vi "CODMn插入数据.vi"(0 "database":string, 1 "data":T2 {"单位" items=["ug/L", "mg/L", "ppm", "mg/m3", "cm", "ppb", "ug/m3", "%", "nmol/mol", "umol/mol", "MPN/L", "MPN/100ml", "ng/m3", "NTU", "无量纲", "ms/cm", "us/cm"]}, 3 "SN":string, 5 "table":string, 7 "测量模式":T3(ring)=enum."水样测试", 9 "数据类型":string(combo)="N", 11 "error in (no error)":errorcluster) -> (15 "error out":errorcluster)   [LabVIEW 2016, in "斯坦道CODMn新电路板.lvlib"]
uses:
  <vilib>/Utility/sysdir.llb/System Directory Type.ctl
  <vilib>/Utility/error.llb/DialogType.ctl
  <vilib>/addons/database/Auxilliary.llb/DB Tools Column Info.ctl
  <vilib>/addons/database/Auxilliary.llb/DB Tools DataTypes.ctl
  <vilib>/addons/database/Connection.llb/DB Tools Open Connec (String).vi
  <vilib>/addons/database/Connection.llb/Conn Execute.vi
  <vilib>/addons/database/Recordset.llb/Rec Fetch Recordset Data (R).vi
  <vilib>/addons/database/Recordset.llb/Rec Destroy - Connection.vi
  <vilib>/addons/database/NI_Database_API.lvlib
  <vilib>/Utility/VariantDataType/VariantType.lvlib
panel:
  out "data输出":T1
  out "为空？":bool
  out "recordset data":variant[][](array[variant])
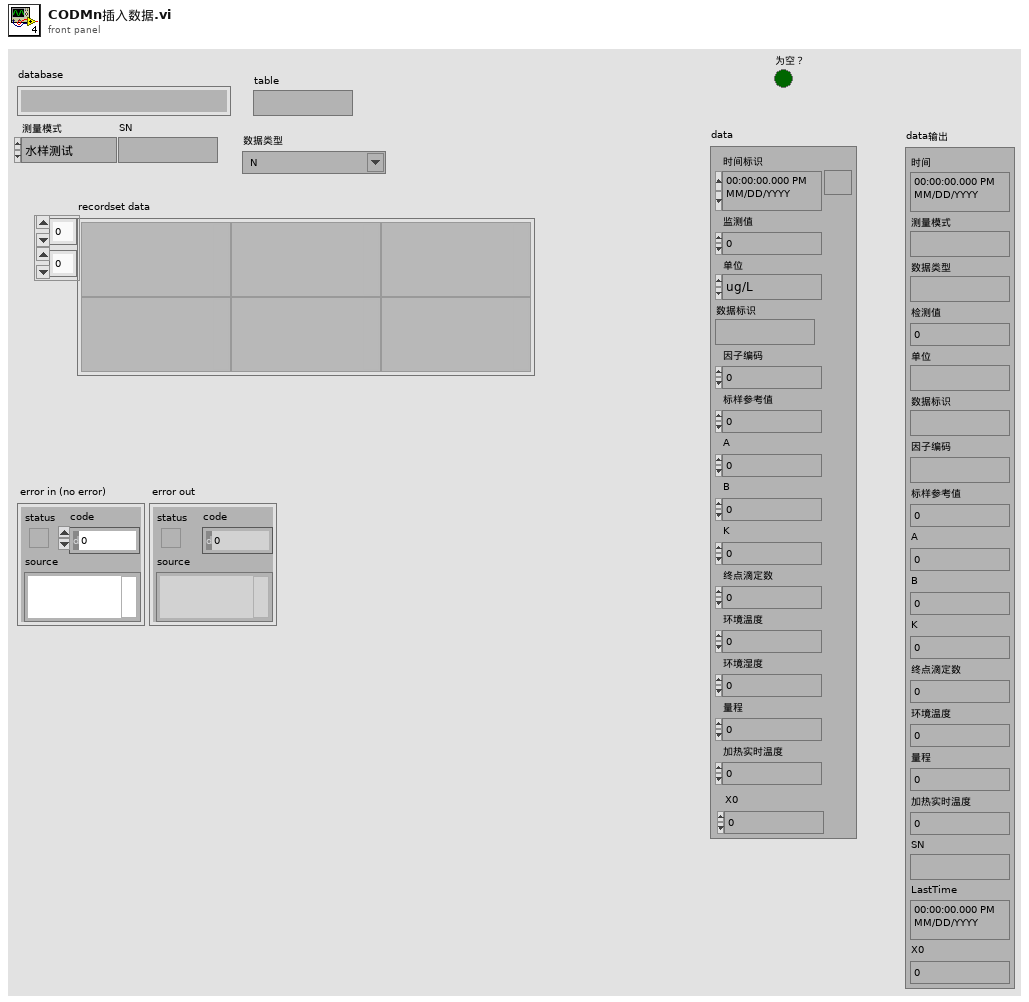
[diagram p1: front panel]
types:
  T1 = cluster{"时间":timestamp, "测量模式":string, "数据类型":string, "检测值":sgl, "单位":string, "数据标识":string, "因子编码":string, "标样参考值":sgl, "A":sgl, "B":sgl, "K":sgl, "终点滴定数":sgl, "环境温度":sgl, "量程":sgl, "加热实时温度":sgl, "SN":string, "LastTime":timestamp, "X0":sgl}
  T2 = cluster{"时间标识":timestamp, "监测值":sgl, "单位":u16, "数据标识":string, "因子编码":u32, "标样参考值":sgl, "A":sgl, "B":sgl, "K":sgl, "终点滴定数":sgl, "环境温度":sgl, "环境湿度":sgl, "量程":sgl, "加热实时温度":sgl, "X0":sgl}
  T3 = enum16{"维护数据", "水样测试", "标样核查", "零点核查", "跨度核查", "空白测试", "平行样测试", "加标回收", "空白校准", "标样校准", "初始化（清洗）"}
  T4 = typedef "DialogType.ctl" = u16
  T5 = typedef "System Directory Type.ctl" = i32
  T6 = typedef "NI_Database_API.lvlib/Conn ObjectReference.ctl" = refnum<k1>
  T7 = typedef "NI_Database_API.lvlib/Rec ObjectReference.ctl" = refnum<k1>
  T8 = typedef "NI_Database_API.lvlib/DB Tools Column Info.ctl" = cluster{"column name":string, "data type":T9, "size":i32, "allow null?":bool}
  T9 = typedef "NI_Database_API.lvlib/DB Tools DataTypes.ctl" = enum16{"String", "Long (I32)", "Single (SGL)", "Double (DBL)", "Date/Time", "Binary"}
  T10 = cluster{"测量量程":dbl, "测量精度":dbl, "测量间隔":dbl, "消解温度":dbl, "消解时长":dbl, "空白校准时间":timestamp, "曲线截距":dbl, "曲线斜率":dbl, "测量检出限":dbl, "测量信号值":dbl, "线性相关系数":dbl, "二次多项式系数":dbl, "标样校准时间":timestamp, "稀释倍数":dbl, "三项式系数":dbl, "空白标定系数":dbl, "量程系数":dbl, "F0/ORPA":dbl, "F1/ORPB":dbl, "F2/ORPK":dbl, "F3":dbl, "F4":dbl, "F5":dbl, "F6":dbl, "F7":dbl, "X0/滴定数":dbl, "量程":dbl}
  T11 = typedef "VariantType.lvlib/Type.ctl" = enum8{"Invalid Type", "Void", "I8", "I16", "I32", "I64", "U8", "U16", "U32", "U64", "Single Float", "Double Float", "Extended Float", "Single Complex", "Double Complex", "Extended Complex", "Enum U8", "Enum U16", "Enum U32", "Enum U64", "Single Float With Unit", "Double Float With Unit", "Extended Float With Unit", "Single Complex with Unit", "Double Complex with Unit", "Extended Complex with Unit", "Boolean", "String", "Path", "Picture", "Tag", "Array", "Cluster", "Variant", "LV Variant", "Waveform", "Timestamp", "Digital Waveform", "Digital Data", "ExpressData", "Refnum", "External Data", "VI", "Poly VI", "LabVIEW Class Instance", "Fixed Point"}
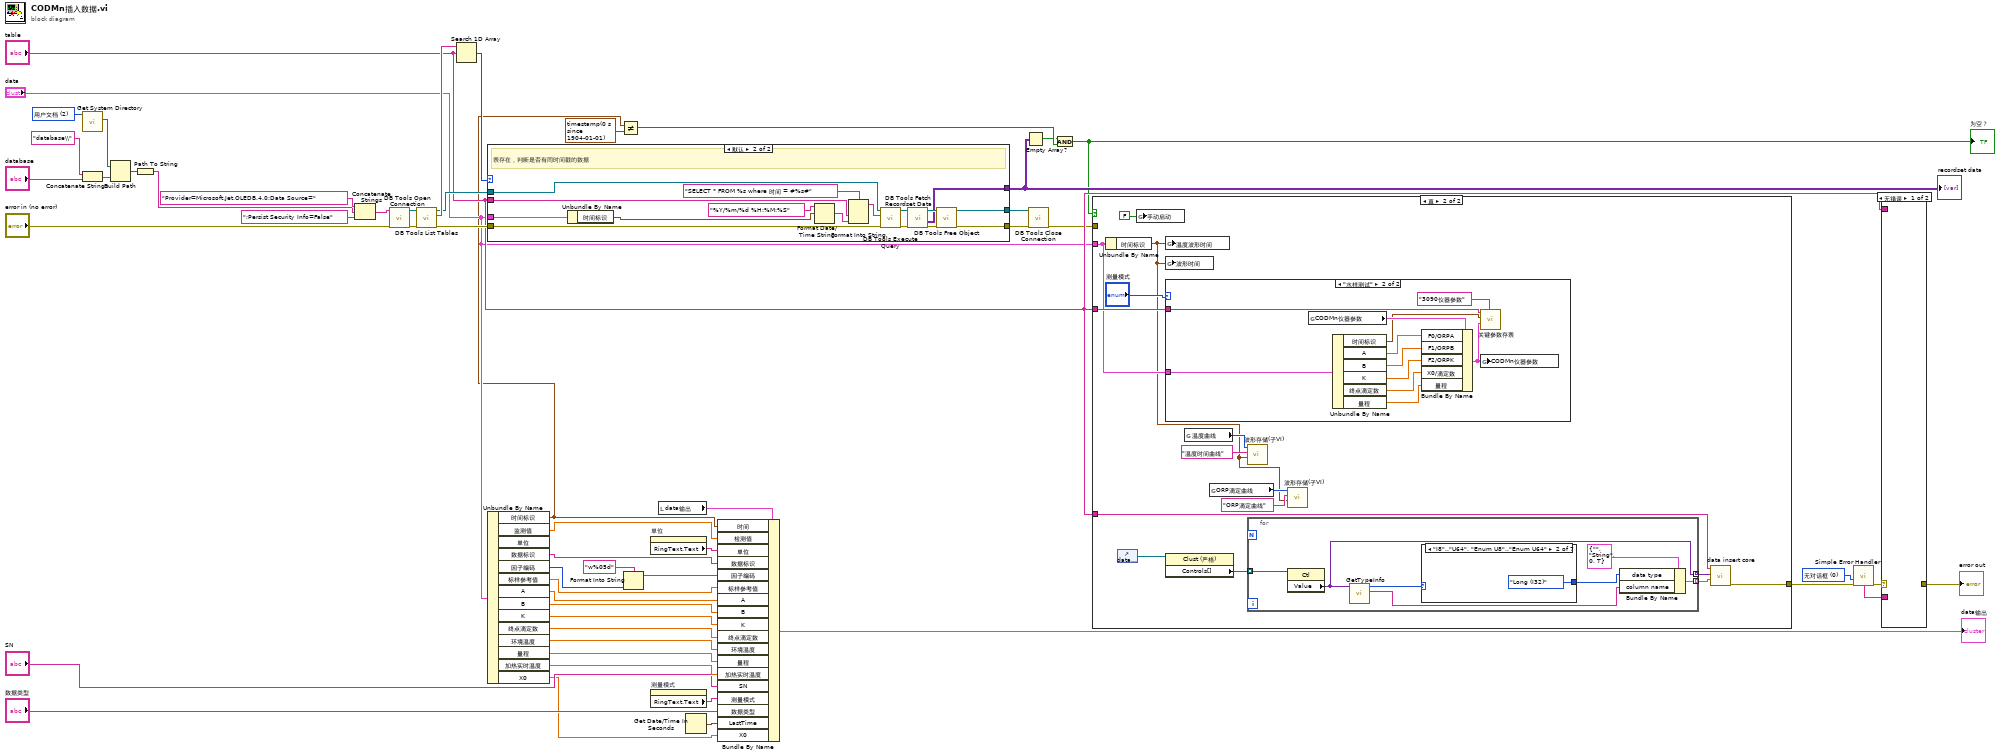
[diagram p0: block diagram]
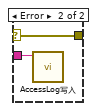
[diagram p2: hidden frame]
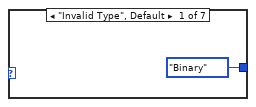
[diagram p4: hidden frame]
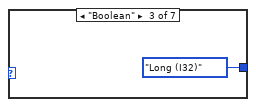
[diagram p5: hidden frame]
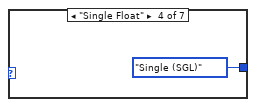
[diagram p6: hidden frame]
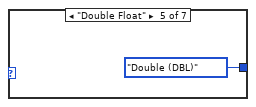
[diagram p7: hidden frame]
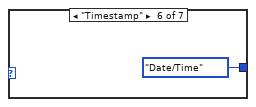
[diagram p8: hidden frame]
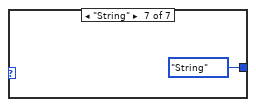
[diagram p9: hidden frame]
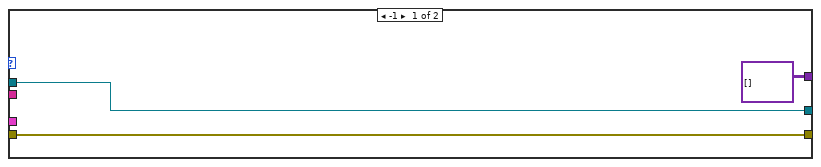
[diagram p11: hidden frame]
diagram:
  w36 = T4 0 items=["无对话框", "确定信息", "继续或停止信息", "确定信息＋警告", "继续/停止+警告"] ("type of dialog (OK msg:1)")
  w53 = T5 2 items=["用户目录"=0, "用户桌面"=1, "用户文档"=2, "用户应用程序数据"=3, "用户设置"=4, "用户临时目录"=5, "公共文档"=6, "公共应用程序数据"=7, "公共设置"=8, "公共缓存"=13, "系统核心库"=9, "系统安装库"=10, "应用程序文件"=11, "启动盘根目录"=12] ("system directory type")
  n1 = call <vilib>:"Get System Directory.vi"("system directory type"=w53) -> ("system directory"=w51:path)  [unwired: 10 in]
  n2 = Concatenate Strings("database\\" ("condition"), "database") -> (w45:string)
  n3 = Build Path(base path=w51, name or relative path=w45) -> (appended path=w50:path)
  n4 = Path To String(path=w50) -> (string=w49:string)
  n5 = Concatenate Strings("Provider=Microsoft.Jet.OLEDB.4.0;Data Source=" ("condition"), w49, ";Persist Security Info=False" ("condition")) -> (w47:string)
  n6 = call-poly <vilib>:"DB Tools Open Connection.vi"("error in (no error)"="error in (no error)", "connection information"=w47) -> ("error out"=w42:errorcluster, "connection reference"=w43:T6)  [unwired: 6 in]
  n7 = call <vilib>:"DB Tools List Tables.vi"("error in (no error)"=w42, "connection reference"=w43) -> ("error out"=w37:errorcluster, "tables"=w41:string[], "connection reference out"=w38:T6)  [unwired: 3 in]
  n8 = Search 1D Array(1D array=w41, element="table") -> (index of element=w40:i32)  [unwired: 1 in]
  n9 = case shown="默认" w40 {
    tunnel: [variant[][] [] ("recordset data") w69] -> w44
    tunnel: [w57 w68] -> w31
    tunnel: [w56 w67] -> w30
    tunnel: w38 -> [w57 w61]
    tunnel: w37 -> [w56 w60]
    tunnel: "table" -> [_ w59]
    tunnel: "data" -> [_ w62]
    frame -1 {
    }
    frame Default {
      # "表存在，判断是否有同时间戳的数据"
      n10 = Unbundle By Name(w62) -> ("时间标识"=w65:timestamp)
      n11 = Format Date/Time String(time format string (%c)="%Y/%m/%d %H:%M:%S" ("时间格式字符串(%c)"), seconds (now)=w65) -> (date/time string=w63:string)  [unwired: 1 in]
      n12 = Format Into String(format string="SELECT * FROM %s where 时间 = #%s#" ("格式字符串"), w59, w63) -> (resulting string=w66:string)  [unwired: 2 in, 1 out]
      n13 = call-poly <vilib>:"DB Tools Execute Query.vi"("error in (no error)"=w60, "SQL query"=w66, "connection reference"=w61) -> ("error out"=w70:errorcluster, "recordset reference"=w73:T7)  [unwired: 5 in]
      n14 = call-poly <vilib>:"DB Tools Fetch Recordset Data.vi"("error in (no error)"=w70, "recordset reference"=w73) -> ("error out"=w71:errorcluster, "recordset data"=w69:variant[][], "recordset reference out"=w72:T7)  [unwired: 3 in]
      n15 = call-poly <vilib>:"DB Tools Free Object.vi"("error in (no error)"=w71, "recordset reference"=w72) -> ("error out"=w67:errorcluster, "connection reference"=w68:T6)  [unwired: 8 in]
    }
  }
  "recordset data" <- w44
  n16 = Unbundle By Name("data") -> ("时间标识"=w5:timestamp, "监测值"=w25:sgl, "数据标识"=w23:string, "因子编码"=w21:u32, "标样参考值"=w19:sgl, "A"=w18:sgl, "B"=w17:sgl, "K"=w16:sgl, "终点滴定数"=w15:sgl, "环境温度"=w14:sgl, "量程"=w13:sgl, "加热实时温度"=w12:sgl, "X0"=w7:sgl)  [unwired: 1 out]
  n17 = Not Equal?(x=w5, y=timestamp(0 s since 1904-01-01)) -> (x != y?=w3:bool)
  n18 = Format Into String(format string="w%05d" ("格式字符串"), w21) -> (resulting string=w20:string)  [unwired: 2 in, 1 out]
  n19 = property on="单位" class="Ring (严格)"() -> ("RingText.Text"=w24:string)  [unwired: 2 in, 2 out]
  n20 = property on="测量模式" class="Enum (严格)"() -> ("RingText.Text"=w10:string)  [unwired: 2 in, 2 out]
  n21 = local read "data输出"() -> (w28:T1)
  n22 = Get Date/Time In Seconds() -> (seconds since 1Jan1904=w8:timestamp)
  n23 = Bundle By Name(cluster=w28, "时间"=w5, "检测值"=w25, "单位"=w24, "数据标识"=w23, "因子编码"=w20, "标样参考值"=w19, "A"=w18, "B"=w17, "K"=w16, "终点滴定数"=w15, "环境温度"=w14, "量程"=w13, "加热实时温度"=w12, "SN"="SN", "测量模式"=w10, "数据类型"="数据类型", "LastTime"=w8, "X0"=w7) -> (→"data输出":T1)
  n24 = Empty Array?(array=w44) -> (empty?=w2:bool)
  n25 = call <vilib>:"DB Tools Close Connection.vi"("error in (no error)"=w30, "connection reference"=w31) -> ("error out"=w29:errorcluster)  [unwired: 5 in]
  n26 = And(x=w2, y=w3) -> (x .and. y?=w1:bool)
  "为空？" <- w1
  n27 = case shown="真" w1 {
    tunnel: "table" -> [_ w75]
    tunnel: "data" -> [_ w86]
    tunnel: w29 -> [_ _]
    tunnel: "table" -> [_ w88]
    tunnel: [_ w74] -> w6
    frame False {
    }
    frame True {
      n28 = Unbundle By Name(w86) -> ("时间标识"=w81:timestamp)
      n29 = control-ref of="data输出"() -> (w79:refnum<vi>)
      n30 = global write "VARCODMn全局变量.vi" "手动启动"(FALSE ("手动启动")) -> ()
      n31 = global write "VARCODMn全局变量.vi" "温度波形时间"(w81) -> ()
      n32 = global write "VARCODMn全局变量.vi" "波形时间"(w81) -> ()
      n33 = case shown="\"水样测试\"" "测量模式" {
        tunnel: w86 -> [_ w112]
        tunnel: w88 -> [_ w110]
        frame "维护数据", Default {
        }
        frame "水样测试" {
          n34 = global read "CODMn断电保存全局变量.vi" "CODMn仪器参数"() -> (w113:T10)
          n35 = Unbundle By Name(w112) -> ("时间标识"=w104:timestamp, "A"=w109:sgl, "B"=w108:sgl, "K"=w107:sgl, "终点滴定数"=w106:sgl, "量程"=w105:sgl)
          n36 = Bundle By Name(cluster=w113, "F0/ORPA"=w109, "F1/ORPB"=w108, "F2/ORPK"=w107, "X0/滴定数"=w106, "量程"=w105) -> (w103:T10)
          n37 = call "关键参数存表.vi"("table"="3090仪器参数", "仪器参数"=w103, "datatime"=w104, "仪器名称"=w110) -> ()  [unwired: 7 in, 1 out]
          n38 = global write "CODMn断电保存全局变量.vi" "CODMn仪器参数"(w103) -> ()
        }
      }
      n39 = property class="Clust (严格)"(reference=w79) -> ("Controls[]"=w77:refnum<vi>[])  [unwired: 1 in, 2 out]
      n40 = global read "VARCODMn全局变量.vi" "温度曲线"() -> (w83:u16[])
      n41 = global read "VARCODMn全局变量.vi" "ORP滴定曲线"() -> (w85:u16[])
      n42 = call "波形存储(子VI).vi"("波形时间"=w81, "condition"="温度时间曲线", "ORP滴定曲线"=w83) -> ()  [unwired: 9 in]
      n43 = for {
        tunnel: w77 -> [w95] mode=indexing
        tunnel: [w89] -> w78 mode=indexing
        tunnel: [w90] -> w76 mode=indexing
        n44 = property class="Ctl"(reference=w95) -> ("Value"=w89:variant)  [unwired: 1 in, 2 out]
        n45 = call <vilib>:"GetTypeInfo.vi"("Variant"=w89) -> ("Name"=w93:string, "Type Enum"=w92:T11)  [unwired: 6 in, 3 out]
        n46 = case shown="\"I8\"..\"U64\", \"Enum U8\"..\"Enum U64\"" w92 {
          tunnel: [DB_Tools_DataTypes."Binary" ("data type") DB_Tools_DataTypes."Long (I32)" ("data type") DB_Tools_DataTypes."Long (I32)" ("data type") DB_Tools_DataTypes."Single (SGL)" ("data type") DB_Tools_DataTypes."Double (DBL)" ("data type") DB_Tools_DataTypes."Date/Time" ("data type") DB_Tools_DataTypes."String" ("data type")] -> w91
          frame "Invalid Type", Default {
          }
          frame "I8".."U64", "Enum U8".."Enum U64" {
          }
          frame "Boolean" {
          }
          frame "Single Float" {
          }
          frame "Double Float" {
          }
          frame "Timestamp" {
          }
          frame "String" {
          }
        }
        n47 = Bundle By Name(cluster=T8 {"column name"="", "data type"=enum."String", "size"=0, "allow null?"=TRUE} ("column information"), "data type"=w91, "column name"=w93) -> (w90:T8)
      }
      n48 = call "波形存储(子VI).vi"("波形时间"=w81, "condition"="ORP滴定曲线", "ORP滴定曲线"=w85) -> ()  [unwired: 9 in]
      n49 = call "data insert core.vi"("column information"=w76, "data"=w78, "table"=w75) -> ("error out"=w74:errorcluster)  [unwired: 8 in]
    }
  }
  n50 = call <vilib>:"Simple Error Handler.vi"("type of dialog (OK msg:1)"=w36, "error in (no error)"=w6) -> ("error out"=w35:errorcluster, "message"=w34:string)  [unwired: 3 in, 3 out]
  n51 = case shown="无错误" w35 {
    selector: w35 -> [_ w114]
    tunnel: w34 -> [_ w115]
    tunnel: [_ w114] -> w33
    tunnel: "table" -> [_ _]
    frame No Error {
    }
    frame Error {
      n52 = call "AccessLog写入.vi"("Log"=w115) -> ()  [unwired: 11 in]
    }
  }
  "error out" <- w33
